vi "getModelInfo.vi"(0 "VISA resource name":refnum<visa-resource-name>, 11 "error in (no error)":errorcluster) -> (4 "VISA resource name out":refnum<visa-resource-name>, 6 "Model Names":string[](array[string]), 8 "Microstep Sizes":dbl[](array[numeric]), 10 "Device Number & Axis":string[](array[string]), 14 "Motion Type":string[](array[string]), 15 "error out":errorcluster)   [LabVIEW 2020]
uses:
  <vilib>/Utility/file.llb/Read Delimited Spreadsheet (string).vi
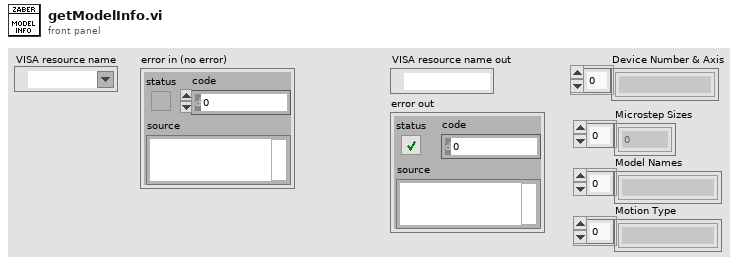
[diagram p1: front panel]
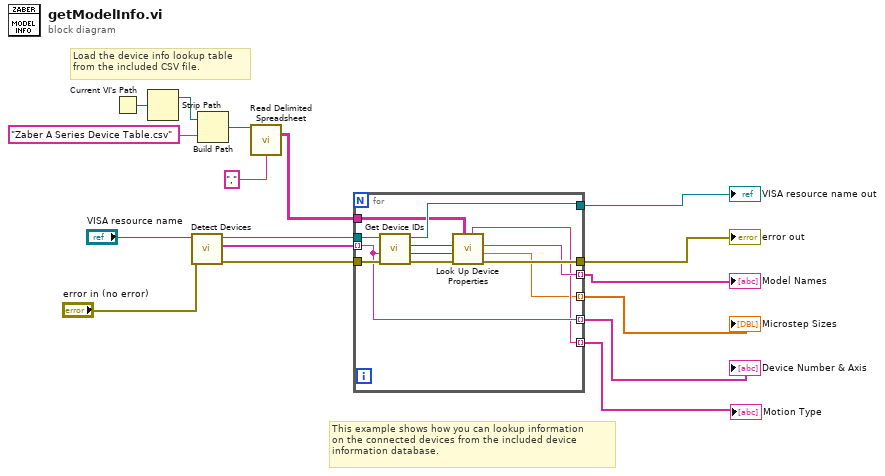
[diagram p0: block diagram]
diagram:
  # "Load the device info lookup table\nfrom the included CSV file."
  # "This example shows how you can lookup information\non the connected devices from the included device \ninformation database."
  n1 = Current VI's Path() -> (path=w9:path)
  n2 = Strip Path(path=w9) -> (stripped path=w10:path)  [unwired: 1 out]
  n3 = call "Detect Devices.vi"("error in (no error)"="error in (no error)", "VISA resource name"="VISA resource name") -> ("error out"=w12:errorcluster, "Connected Devices and Axes"=w13:string[], "VISA resource name out"=w11:refnum<visa-resource-name>)  [unwired: 6 in, 1 out]
  n4 = Build Path(base path=w10, name or relative path="Zaber A Series Device Table.csv") -> (appended path=w7:path)
  n5 = call-poly <vilib>:"Read Delimited Spreadsheet.vi"("file path (dialog if empty)"=w7, "delimiter (\\t)"="," ("delimiter (\\t)")) -> ("all rows"=w5:string[][])  [unwired: 8 in, 5 out]
  n6 = for {
    tunnel: w11 -> [w29]
    tunnel: w12 -> [w28]
    tunnel: [w24] -> w1
    tunnel: w13 -> [w23] mode=indexing
    tunnel: [w23] -> w14 mode=indexing
    tunnel: [w22] -> w15 mode=indexing
    tunnel: [w18] -> w16 mode=indexing
    tunnel: [w21] -> w17 mode=indexing
    tunnel: [w20] -> w2
    tunnel: w5 -> [w19]
    n7 = call "Get Device IDs.vi"("error in (no error)"=w28, "Device and Axis"=w23, "VISA resource name"=w29) -> ("error out"=w25:errorcluster, "Peripheral ID"=w26:i32, "Device ID"=w27:i32, "VISA resource name out"=w20:refnum<visa-resource-name>)  [unwired: 5 in]
    n8 = call "Look Up Device Properties.vi"("Lookup Table"=w19, "error in (no error)"=w25, "Peripheral ID (0)"=w26, "Device ID"=w27) -> ("error out"=w24:errorcluster, "Microstep Size"=w18:dbl, "Device Name"=w22:string, "Motion Type"=w21:string)  [unwired: 4 in]
  }
  "VISA resource name out" <- w2
  "error out" <- w1
  "Model Names" <- w15
  "Microstep Sizes" <- w16
  "Device Number & Axis" <- w14
  "Motion Type" <- w17
